vi "PPartner.vi"() -> ()   [LabVIEW 2018]
uses:
  lib/Snap7.lvlib
panel:
  out "Data":bool
  out "R_ID":u32 format="%08x"
  out "Size":i32
  out "Data":string
  out "Partner Status":i32(ring) items=["Stopped", "Connecting", "Waiting", "Linked", "Sending", "Receiving", "Bind Error"]
  in  "stop":bool
  in  "TSAP":u16=4098 format="%x"
  in  "Address IP":string="192.168.1.200"
  out "Start Result":string
  in  "TSAP":u16=4098 format="%x"
  in  "Address IP":string="0.0.0.0"
  # "Local"
  # "Remote"
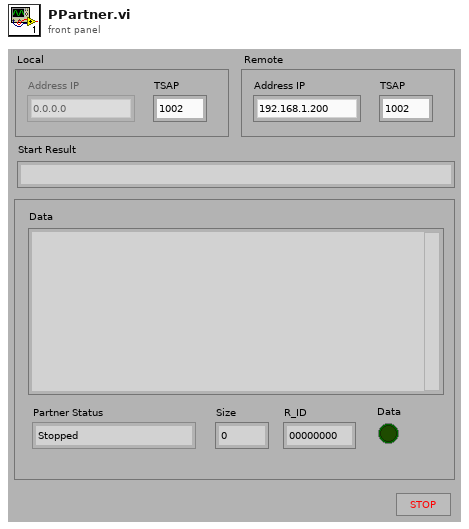
[diagram p1: front panel]
types:
  T1 = enum16{"big-endian, network order", "native, host order", "little-endian"}
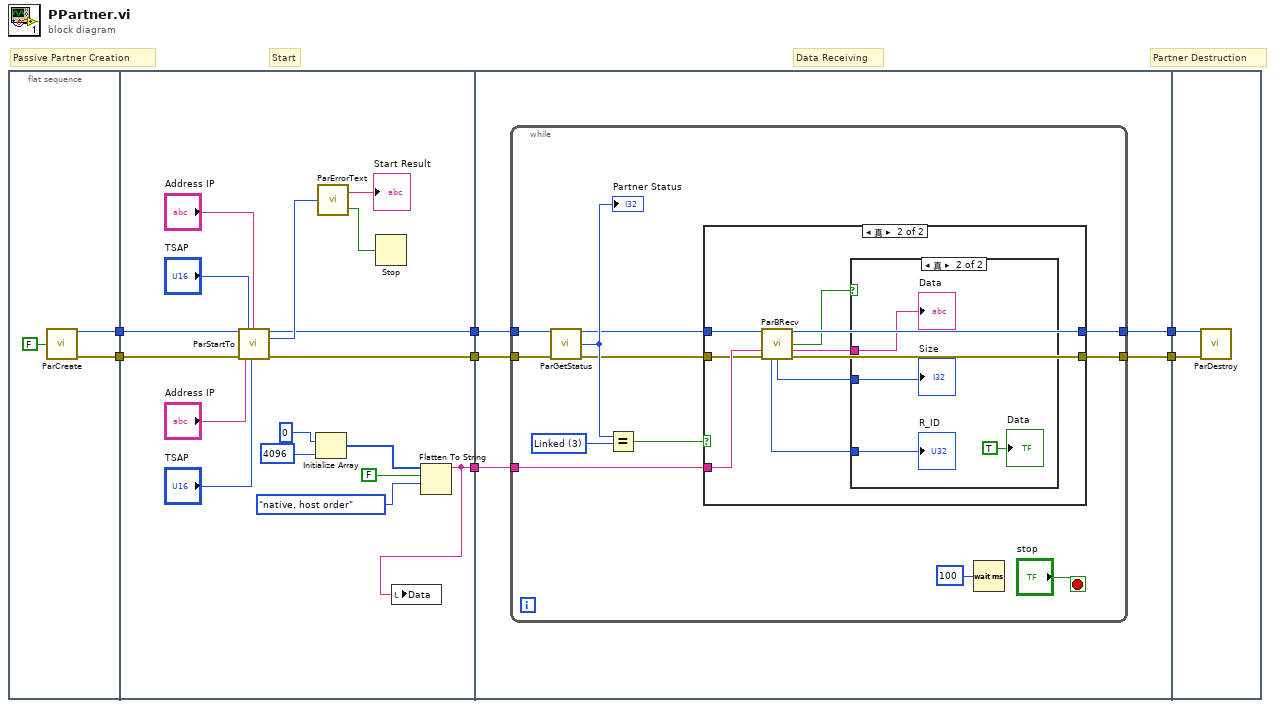
[diagram p0: block diagram]
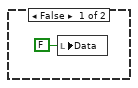
[diagram p3: hidden frame]
diagram:
  # "Partner Destruction"
  # "Data Receiving"
  # "Start"
  # "Passive Partner Creation"
  n1 = flat-sequence {
    tunnel: [w9] -> w7
    tunnel: [w8] -> w6
    tunnel: w7 -> [w25]
    tunnel: w6 -> [w27]
    tunnel: [w18] -> w5
    tunnel: [w17] -> w4
    tunnel: [w11] -> w1
    tunnel: w5 -> [w32]
    tunnel: w4 -> [w31]
    tunnel: [w30] -> w3
    tunnel: [w29] -> w2
    tunnel: w1 -> [w28]
    tunnel: w3 -> [w62]
    tunnel: w2 -> [w61]
    frame #0 {
      n2 = call "ParCreate.vi"("Boolean"=FALSE) -> ("ref out"=w9:u64, "error out"=w8:errorcluster)  [unwired: 13 in]
    }
    frame #1 {
      n3 = call "ParStartTo.vi"("ref in"=w25, "LocalTSAP"="TSAP", "Local Address"="Address IP", "error in (no error)"=w27, "Remote Address"="Address IP", "RemoteTSAP"="TSAP") -> ("ref out"=w18:u64, "Result"=w19:i32, "error out"=w17:errorcluster)  [unwired: 7 in]
      n4 = Initialize Array(u8 0, 4096) -> (w14:u8[])
      n5 = call "ParErrorText.vi"("ErrNo"=w19) -> ("Error"=w20:bool, "ErrMessage"=→"Start Result":string)
      n6 = Stop(stop? (T)=w20) -> ()
      n7 = Flatten To String(anything=w14, prepend array or string size? (T)=FALSE, byte order (0:big-endian, network order)=T1."native, host order") -> (data string=w11:string)  [unwired: 1 in, 2 out]
      n8 = local write "Data"(w11) -> ()
    }
    frame #2 {
      n9 = while {
        tunnel: w32 -> [w43]
        tunnel: w31 -> [w42]
        tunnel: [w36] -> w30
        tunnel: [w33] -> w29
        tunnel: w28 -> [w35]
        stop <- "stop" stop-if-true
        w40 = 3 items=["Stopped", "Connecting", "Waiting", "Linked", "Sending", "Receiving", "Bind Error"] ("Partner Status 2")
        n10 = call "ParGetStatus.vi"("ref in"=w43, "error in (no error)"=w42) -> ("ref out"=w37:u64, "Status"=w39:i32, "error out"=w34:errorcluster)  [unwired: 10 in, 1 out]
        "Partner Status" <- w39
        n11 = Equal?(x=w39, y=w40) -> (x = y?=w38:bool)
        n12 = case shown="真" w38 {
          tunnel: w37 -> [w46 w55]
          tunnel: [w46 w54] -> w36
          tunnel: w35 -> [_ w53]
          tunnel: w34 -> [w45 w52]
          tunnel: [w45 w51] -> w33
          frame False {
          }
          frame True {
            n13 = call "ParBRecv.vi"("ref in"=w55, "data in"=w53, "error in (no error)"=w52) -> ("ref out"=w54:u64, "DataReady"=w50:bool, "data out"=w49:string, "R_ID"=w47:u32, "Size"=w48:i32, "error out"=w51:errorcluster)  [unwired: 6 in, 1 out]
            n14 = case shown="真" w50 {
              tunnel: w49 -> [_ w60]
              tunnel: w48 -> [_ w59]
              tunnel: w47 -> [_ w58]
              frame False {
                n15 = local write "Data"(FALSE ("Data")) -> ()
              }
              frame True {
                "Data" <- w60
                "Size" <- w59
                "R_ID" <- w58
                "Data" <- TRUE ("Data")
              }
            }
          }
        }
        n16 = Wait (ms)(milliseconds to wait=u32 100 ("Loop Delay (ms)")) -> ()  [unwired: 1 out]
      }
    }
    frame #3 {
      n17 = call "ParDestroy.vi"("ref in"=w62, "error in (no error)"=w61) -> ()  [unwired: 13 in, 1 out]
    }
  }
